vi "Frame_to_word_Felica UP.vi"() -> ()   [LabVIEW 2019]
uses:
  <vilib>/addons/Modulation/Analog/MT Modulate AM (DSB).vi
  <vilib>/addons/Modulation/Analog/MT Upconvert Baseband (Real).vi
  <vilib>/express/express analysis/Spectral/Block/exnSpectralBlock spectral measurements RMS poly.vi
  <vilib>/express/express analysis/Spectral/Block/exnSpectralBlock spectral measurements RMS WFM.vi
  <vilib>/ErrorRing/Error Ring.xnode
  <vilib>/express/express analysis/Spectral/XNode/ExpressSpectralMeasurementsBlockNode.xnode
  <vilib>/addons/Modulation/niAMT.lvlib
panel:
  out "video Manchecter 2":cluster{"t0":dbl, "dt":dbl, "Y":dbl[]}(graph)
  out "30% OOK":waveform(dbl)(graph)
  out "video Manchecter":cluster{"t0":dbl, "dt":dbl, "Y":dbl[]}(graph)
  in  "BIT RATE":dbl
  in  "CARRIER (hz)":dbl
  out "Video  without CRC":cluster{"t0":dbl, "dt":dbl, "Y":dbl[]}(graph)
  out "Video":cluster{"t0":dbl, "dt":dbl, "Y":dbl[]}(graph)
  in  "Preambul":u8[](array[numeric])=[0, 0, 0, 0, 0, 0] format="%x"
  in  "SYNC":u8[](array[numeric])=[178, 212] format="%x"
  in  "DID":u8[](array[numeric])=[20] format="%x"
  in  "CMD2":u8[](array[numeric])=[3] format="%x"
  in  "CMD1":u8[](array[numeric])=[213] format="%x"
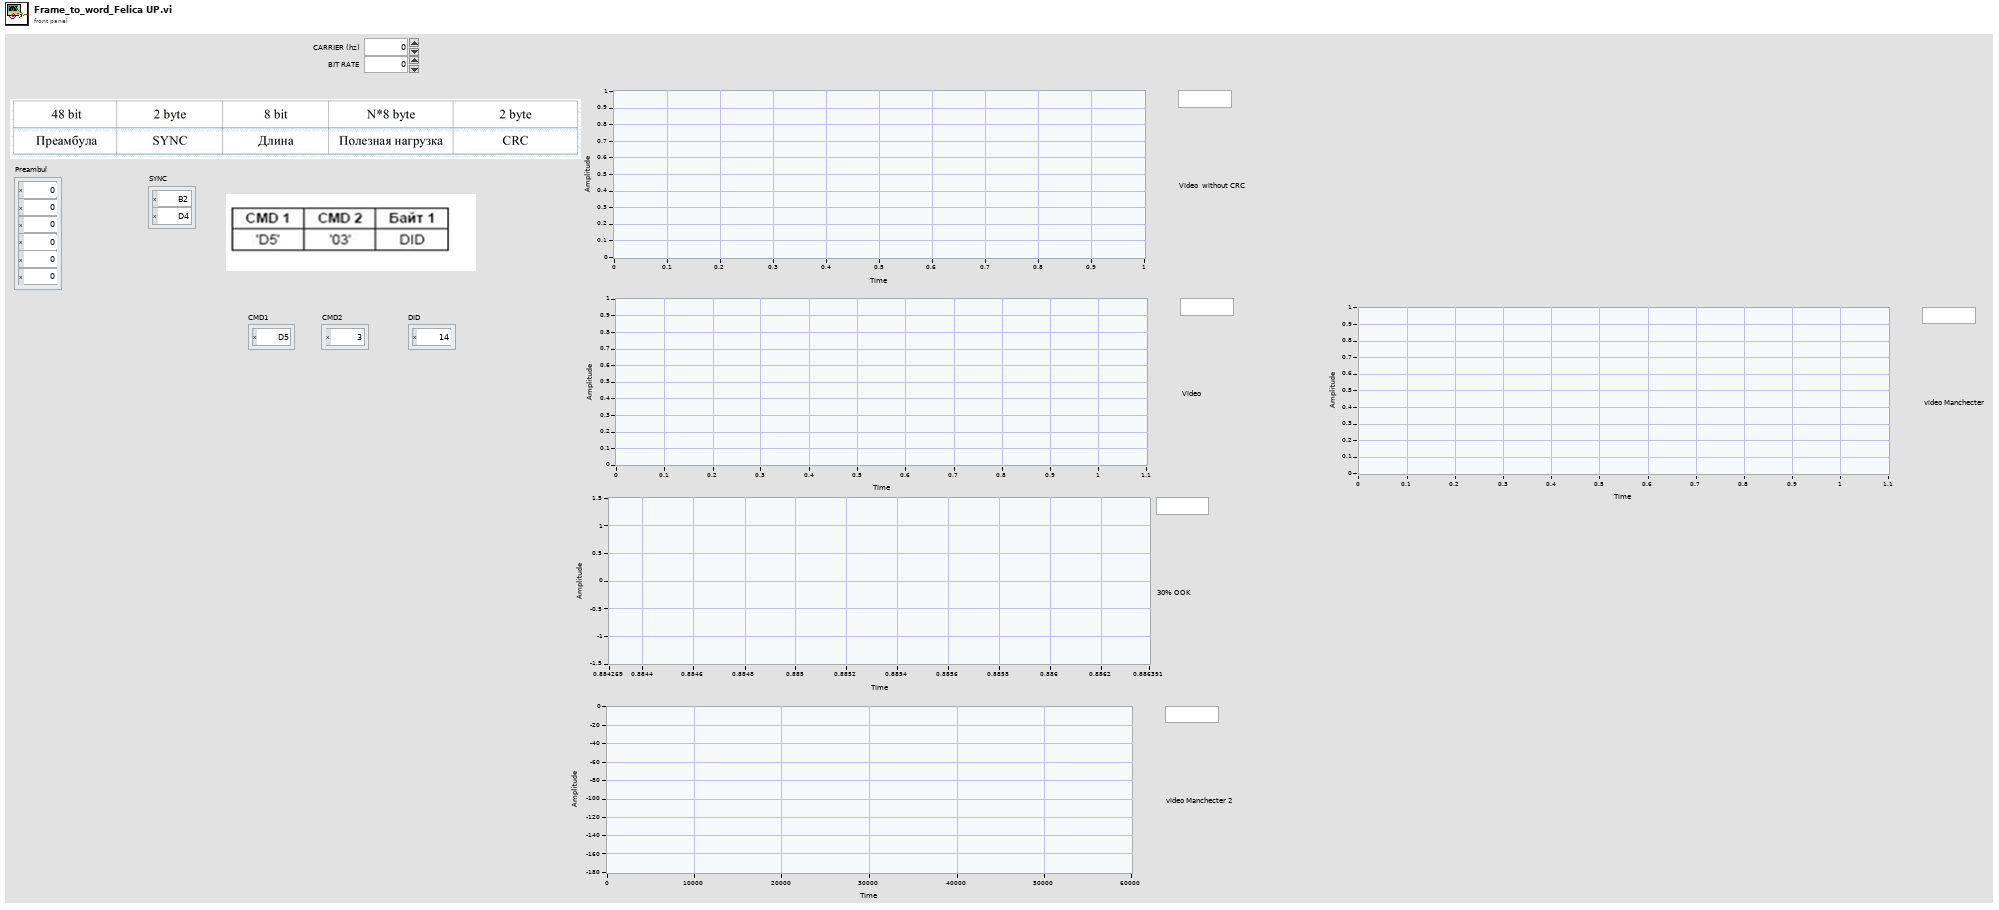
[diagram p1: front panel]
types:
  T1 = typedef "niAMT.lvlib/Complex Data Waveform.ctl" = cluster{"t0":dbl, "dt":dbl, "Y":cdb[]}
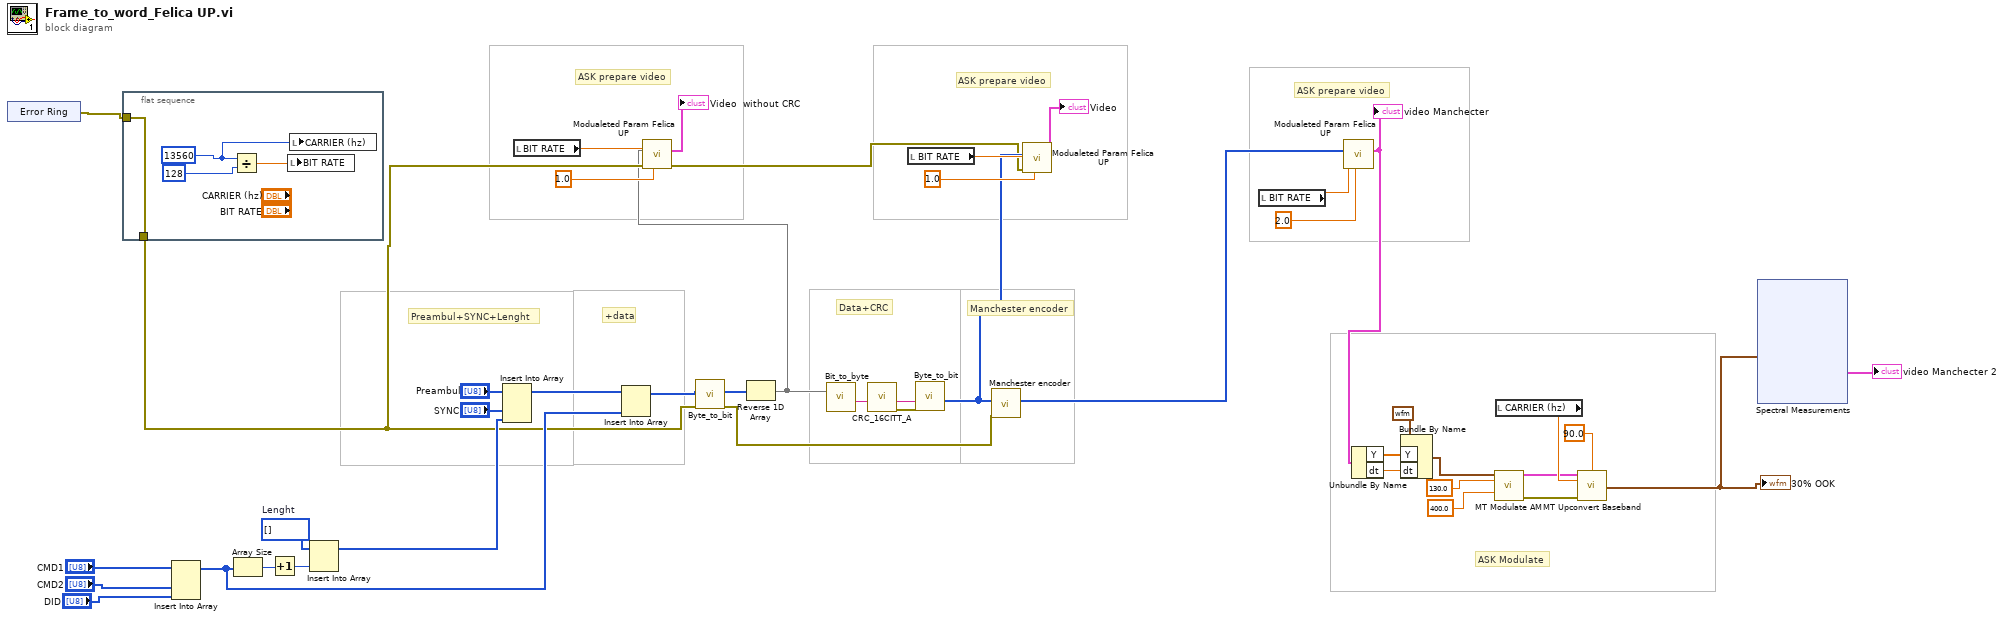
[diagram p0: block diagram]
diagram:
  w39 = u8[] []  # Lenght
  # "ASK Modulate"
  # "ASK prepare video"
  # "ASK prepare video"
  # "ASK prepare video"
  # "Manchester encoder"
  # "Data+CRC"
  # "+data"
  # "Preambul+SYNC+Lenght"
  n1 = xnode "Error Ring"() -> ("error out"=w22:errorcluster)
  n2 = flat-sequence {
    tunnel: w22 -> [w45]
    tunnel: [w45] -> w21
    frame #0 {
      w46 = u32 13560
      n3 = Divide(x=w46, y=u32 128) -> (x/y=w47:dbl)
      n4 = local write "BIT RATE"(w47) -> ()
      n5 = local write "CARRIER (hz)"(w46) -> ()
    }
  }
  n6 = Insert Into Array(array="CMD1", new element #1="CMD2", new element #2="DID") -> (w35:u8[])  [unwired: 1 in]
  n7 = Array Size(array=w35) -> (size(s)=w41:i32)
  n8 = Increment(x=w41) -> (x+1=w40:i32)
  n9 = Insert Into Array(array=w39, new element=w40) -> (w36:u8[])  [unwired: 1 in]
  n10 = Insert Into Array(array="Preambul", new element #1="SYNC", new element #2=w36) -> (w34:u8[])  [unwired: 1 in]
  n11 = local read "BIT RATE"() -> (w27:dbl)
  n12 = Insert Into Array(array=w34, new element=w35) -> (w25:u8[])  [unwired: 1 in]
  n13 = call "Byte_to_bit.vi"("Error In"=w21, "Array of byte"=w25) -> ("Error Out"=w23:errorcluster, "Arrray of bit"=w24:u8[])  [unwired: 5 in, 1 out]
  n14 = Reverse 1D Array(array=w24) -> (reversed array=w19:u8[])
  n15 = call "Modualeted Param Felica UP.vi"("encoder divider"=1.0 ("y"), "Error In"=w21, "BIT RATE"=w27, "Bit stream out (NRZ encode)"=w19) -> ("Error Out"=w20:errorcluster, "output complex waveform"=→"Video  without CRC":T1)  [unwired: 6 in]
  n16 = call "Bit_to_byte.vi"("Array of bit"=w19) -> ("BYTE"=w2:string)  [unwired: 8 in, 2 out]
  n17 = call "CRC_16CITT_A.vi"("DATA PACKET"=w2) -> ("Error Out"=w33:errorcluster, "DATA PACKET+CRC"=w1:string)  [unwired: 6 in, 1 out]
  n18 = local read "BIT RATE"() -> (w32:dbl)
  n19 = call "Byte_to_bit.vi"("Error In"=w33, "BYTE"=w1) -> ("Arrray of bit (str)"=w26:u8[])  [unwired: 5 in, 2 out]
  n20 = call "Manchester encoder.vi"("Error In"=w23, "Bit stream in"=w26) -> ("Bit stream out (Manchester encode)"=w16:u8[])  [unwired: 8 in, 1 out]
  n21 = call "Modualeted Param Felica UP.vi"("encoder divider"=1.0 ("y"), "Error In"=w20, "BIT RATE"=w32, "Bit stream out (NRZ encode)"=w26) -> ("output complex waveform"=→"Video":T1)  [unwired: 6 in, 1 out]
  n22 = local read "BIT RATE"() -> (w17:dbl)
  n23 = call "Modualeted Param Felica UP.vi"("encoder divider"=2.0 ("y"), "BIT RATE"=w17, "Bit stream out (NRZ encode)"=w16) -> ("output complex waveform"=w6:T1)  [unwired: 7 in, 1 out]
  "video Manchecter" <- w6
  n24 = Unbundle By Name(w6) -> ("Y"=w13:cdb[], "dt"=w3:dbl)
  n25 = Bundle By Name(cluster=waveform(cdb) {"t0"=timestamp(0 s since 1904-01-01), "dt"=1.0, "Y"=[]} ("waveform"), "Y"=w13, "dt"=w3) -> (w10:waveform(cdb))
  n26 = call-poly <vilib>:"MT Modulate AM.vi"("message signal"=w10, "modulation index"=130.0, "peak message amplitude"=400.0) -> ("AM modulated waveform"=w11:cluster{"t0":dbl, "dt":dbl, "Y":cdb[]}, "error out"=w8:errorcluster)  [unwired: 11 in]
  n27 = local read "CARRIER (hz)"() -> (w12:dbl)
  n28 = call-poly <vilib>:"MT Upconvert Baseband.vi"("baseband waveform (complex)"=w11, "initial phase (deg)"=90.0, "carrier frequency (Hz)"=w12, "error in (no error)"=w8) -> ("passband waveform"=w5:waveform(dbl))  [unwired: 10 in, 1 out]
  "30% OOK" <- w5
  n29 = xnode "Spectral Measurements"("Signals"=w5) -> ("FFT - (RMS)"=→"video Manchecter 2":cluster{"f0":dbl, "df":dbl, "magnitude":dbl[]})  [unwired: 1 in, 2 out]
